vi "PH_uOPA_DelayController.PC set Feedback Control.vi"(0 "VI in":refnum<vi>, 2 "Feedback Control":bool, 5 "error in (no error)":errorcluster) -> (14 "VI out":refnum<vi>, 19 "error out":errorcluster)   [LabVIEW 2014, in "PH_uOPA_DelayController.lvlib"]
uses:
  PH_uOPA_DelayController.lvlib
  PH_Basics/PH_Common/PH_Common.lvlib
  PH_Basics/PH_AxisGUI_BaseClass/PH_AxisGUI_BaseClass.lvlib
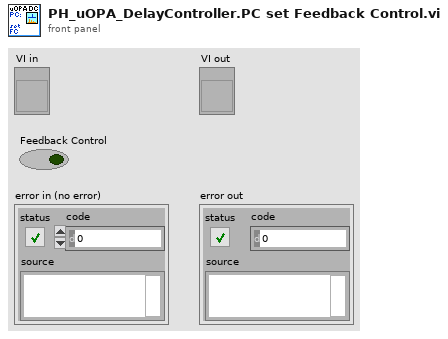
[diagram p1: front panel]
types:
  T1 = typedef "PH_uOPA_DelayController.lvlib/PH_uOPA_DelayController.i attribute.ctl" = cluster{"GUI Refs":cluster{"Current Pump Peak":refnum<vi>, "Current uOPA Peak":refnum<vi>, "Pump Peak":refnum<vi>, "uOPA Peak":refnum<vi>, "uOPA Target":refnum<vi>, "uOPA Limits [%]":refnum<vi>, "sample length":refnum<vi>, "Pump Target":refnum<vi>, "Pump Limit":refnum<vi>, "Pump running":refnum<vi>, "Feedback Control":refnum<vi>, "Control Status":refnum<vi>, "uOPA Mean":refnum<vi>, "Current uOPA Mean":refnum<vi>}, "uOPA Target":dbl, "uOPA Limits [%]":T2, "Sample Length":i32, "Initialize Mean":bool, "Pump Target":dbl, "Pump Limit [%]":dbl, "Feedback Control":bool, "Control Status":T3, "last Mean":dbl, "last direction":T4, "Axis Settings":T5, "Width while feedback":dbl}
  T2 = typedef "PH_uOPA_DelayController.lvlib/PH_uOPA_DelayController.Limit.ctl" = cluster{"low":dbl, "activate":dbl, "fine":dbl}
  T3 = typedef "PH_uOPA_DelayController.lvlib/PH_uOPA_DelayController.Control Status.ctl" = enum32{"off", "Pump off", "calculating", "too low", "activated", "fine"}
  T4 = typedef "PH_Stepmotor_BaseClass.lvlib/PH_Stepmotor_BaseClass.Axis Direction.ctl" = enum16{"forward", "backward"}
  T5 = typedef "PH_Stepmotor_BaseClass.lvlib/PH_Stepmotor_BaseClass.Axis Settings.ctl" = cluster{"Sign change":bool, "Width":dbl, "Calibration":dbl, "Unit":string, "Motor Type":T6, "Unit Width":string, "Unit CF":string}
  T6 = typedef "PH_Stepmotor_BaseClass.lvlib/PH_Stepmotor_BaseClass.Motor Type.ctl" = enum16{"Unspecific", "OWIS 49.120.2633", "OWIS 49.060.1033", "OWIS 43.040.2558", "Diamond Motion 2200 series", "OWIS 49.120.266B.MV6", "Calorimeter", "Linear Stage 1", "MICOS VT-80", "MICOS VT-80 S", "Standa Rotstage nt0.95A", "PUF RA 320.200", "PUF RA 800.200", "PUF RA 800.400", "PUF RA 400.50", "1324.nn.800.50", "1324.n9c.800.50", "1324.nn.320.200", "1324.nn.400.200", "1324.nn.800.200", "1324.nn.400.50", "1324.8c9c.800.50", "1324.8c9c.400.200"}
  T7 = enum8{"Enabled", "Disabled", "Disabled and Grayed Out"}
  T8 = typedef "PH_AxisGUI_BaseClass.lvlib/PH_AxisGUI_BaseClass.i attribute.ctl" = cluster{"Axes":T9[]}
  T9 = typedef "PH_AxisGUI_BaseClass.lvlib/PH_AxisGUI_BaseClass.Axis Attributes.ctl" = cluster{"Axis GUI Refs":T10, "Address":T11, "Name":string, "Label \"Back\"":string, "Labell \"Forth\"":string, "Moving?":bool}
  T10 = typedef "PH_AxisGUI_BaseClass.lvlib/PH_AxisGUI_BaseClass.Axis GUI Refs.ctl" = cluster{"Back":refnum<vi>, "Forth":refnum<vi>, "Status":refnum<vi>, "Target":refnum<vi>, "Address":refnum<vi>, "Status Bar":refnum<vi>, "Settings":refnum<vi>, "Activity":refnum<vi>, "Clear Error":refnum<vi>}
  T11 = typedef "PH_Stepmotor_BaseClass.lvlib/PH_Stepmotor_BaseClass.Axis Address.ctl" = cluster{"Instance":string, "Motor Nr":i32}
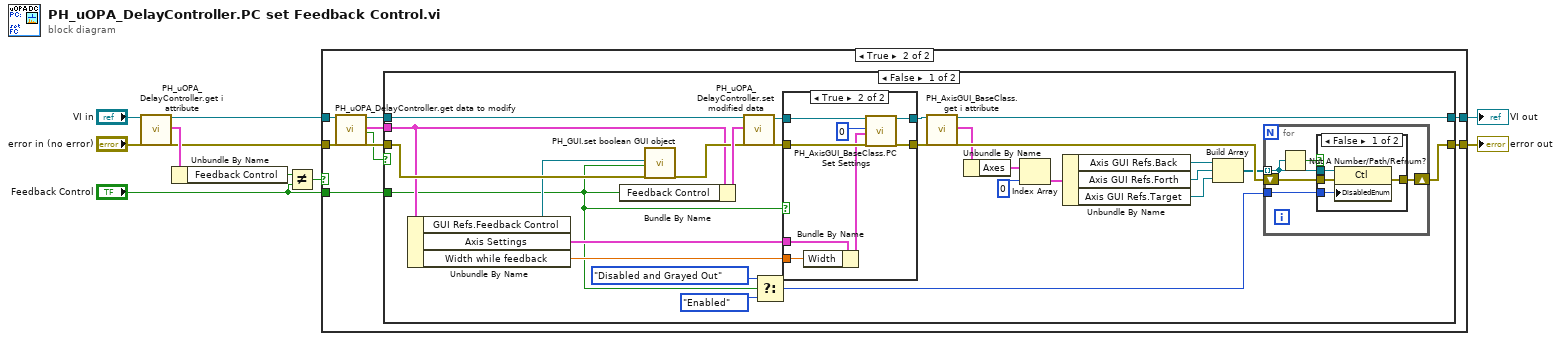
[diagram p0: block diagram]
diagram:
  n1 = call "PH_uOPA_DelayController.get i attribute.vi"("i ref in"="VI in", "error in (no error)"="error in (no error)") -> ("i ref out"=w6:refnum<vi>, "i attribute"=w7:T1, "error out"=w4:errorcluster)  [unwired: 15 in]
  n2 = Unbundle By Name(w7) -> ("Feedback Control"=w8:bool)
  n3 = Not Equal?(x=w8, y="Feedback Control") -> (x != y?=w10:bool)
  n4 = case shown="True" w10 {
    tunnel: [w11 w20] -> w2
    tunnel: [w12 w18] -> w3
    tunnel: w4 -> [w11 w15]
    tunnel: w6 -> [w12 w14]
    tunnel: "Feedback Control" -> [_ w13]
    frame False {
    }
    frame True {
      n5 = call "PH_uOPA_DelayController.get data to modify.vi"("i ref in"=w14, "error in (no error)"=w15) -> ("i ref out"=w19:refnum<vi>, "i attribute"=w16:T1, "timed out"=w17:bool, "error out"=w21:errorcluster)  [unwired: 14 in]
      n6 = case shown="False" w17 {
        tunnel: w21 -> [w48 w69]
        tunnel: [w27 w69] -> w20
        tunnel: w19 -> [w47 w70]
        tunnel: [w35 w70] -> w18
        tunnel: w16 -> [w44 _]
        tunnel: w13 -> [w25 _]
        frame False {
          n7 = Unbundle By Name(w44) -> ("GUI Refs.Feedback Control"=w43:refnum<vi>, "Axis Settings"=w39:T5, "Width while feedback"=w38:dbl)
          n8 = Bundle By Name(cluster=w44, "Feedback Control"=w25) -> (w46:T1)
          n9 = call "PH_GUI.set boolean GUI object.vi"("Boolean Knob GUI Ref"=w43, "Value"=w25, "error in (no error)"=w48) -> ("error out"=w45:errorcluster)  [unwired: 16 in]
          n10 = call "PH_uOPA_DelayController.set modified data.vi"("i ref in"=w47, "i attribute"=w46, "error in (no error)"=w45) -> ("i ref out"=w42:refnum<vi>, "error out"=w41:errorcluster)  [unwired: 15 in]
          n11 = Select(t=T7."Disabled and Grayed Out" ("Disabled"), s=w25, f=T7."Enabled" ("Disabled")) -> (s? t:f=w22:T7)
          n12 = case shown="True" w25 {
            tunnel: w42 -> [w60 w68]
            tunnel: [w60 w67] -> w36
            tunnel: w41 -> [w59 w66]
            tunnel: [w59 w65] -> w40
            tunnel: w39 -> [_ w63]
            tunnel: w38 -> [_ w61]
            frame False {
            }
            frame True {
              n13 = Bundle By Name(cluster=w63, "Width"=w61) -> (w62:T5)
              n14 = call "PH_AxisGUI_BaseClass.PC Set Settings.vi"("VI in"=w68, "Axis"=0, "NewVal"=w62, "error in (no error)"=w66) -> ("VI out"=w67:refnum<vi>, "error out"=w65:errorcluster)  [unwired: 14 in]
            }
          }
          n15 = call "PH_AxisGUI_BaseClass.get i attribute.vi"("i ref in"=w36, "error in (no error)"=w40) -> ("i ref out"=w35:refnum<vi>, "i attribute"=w34:T8, "error out"=w37:errorcluster)  [unwired: 15 in]
          n16 = Unbundle By Name(w34) -> ("Axes"=w33:T9[])
          n17 = Index Array(array=w33, index=0) -> (element=w31:T9)
          n18 = Unbundle By Name(w31) -> ("Axis GUI Refs.Back"=w30:refnum<vi>, "Axis GUI Refs.Forth"=w29:refnum<vi>, "Axis GUI Refs.Target"=w28:refnum<vi>)
          n19 = Build Array(w30, w29, w28) -> (w26:refnum<vi>[])
          n20 = for {
            shift-right: [w52] -> w27
            shift-left: w37 -> [w53]
            tunnel: w26 -> [w49] mode=indexing
            tunnel: w22 -> [w51]
            n21 = Not A Number/Path/Refnum?(number/path/refnum=w49) -> (NaN/Path/Refnum?=w50:bool)
            n22 = case shown="False" w50 {
              tunnel: w53 -> [w57 w58]
              tunnel: [w56 w58] -> w52
              tunnel: w49 -> [w55 _]
              tunnel: w51 -> [w54 _]
              frame False {
                n23 = property class="Ctl"(reference=w55, error in=w57, "DisabledEnum"=w54) -> (error out=w56:errorcluster)  [unwired: 1 out]
              }
              frame True {
              }
            }
          }
        }
        frame True {
        }
      }
    }
  }
  "VI out" <- w3
  "error out" <- w2
